vi "Deviated Result.vi"(8 "Error in":errorcluster, 11 "Device in":refnum<class "Device.lvclass">) -> (0 "Error out":errorcluster, 3 "Device out":refnum<class "Device.lvclass">)   [LabVIEW 2020, in "Device.lvclass"]
doc: "Dynamic method to calculate deviated result"
uses:
  Device.lvclass
  Device.lvclass/Device.ctl
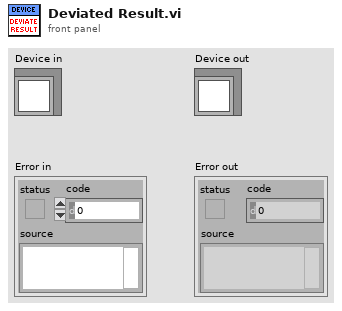
[diagram p1: front panel]
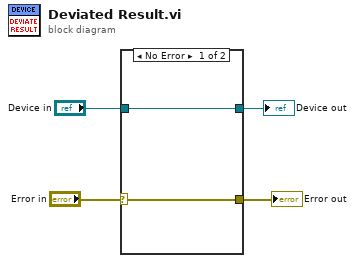
[diagram p0: block diagram]
diagram:
  n1 = case shown="No Error" "Error in" {
    selector: "Error in" -> [w5 w8]
    tunnel: [w5 w8] -> w3
    tunnel: [w6 w7] -> w1
    tunnel: "Device in" -> [w6 w7]
    frame No Error {
    }
    frame Error {
    }
  }
  "Error out" <- w3
  "Device out" <- w1
